vi "FPGA_SviTockovi.vi"() -> ()   [LabVIEW 2014]
uses:
  <vilib>/rvi/Emulation/niFpgaGetClockAttributes.vi
  <vilib>/rvi/Emulation/niFpgaSctlEmulationGetInTimedLoop.vi
  <vilib>/rvi/Emulation/niFpgaEmulationReportErrorSimple.vi
  <vilib>/rvi/eio/common/nirviEmuTemplateMethod_errors.vi
  <vilib>/rvi/Emulation/niFpgaCriticalErrorInLSC.vi
  <vilib>/eio/EIONode/EIONode.xnode
panel:
  in  "stop":bool
  in  "step":sgl(knob) scale=0.0..300.0
  in  "rezolucija":i32(listbox)
  in  "pokreni":bool
  in  "dir 4":bool
  in  "dir 3":bool
  in  "dir 2":bool
  in  "dir 1":bool
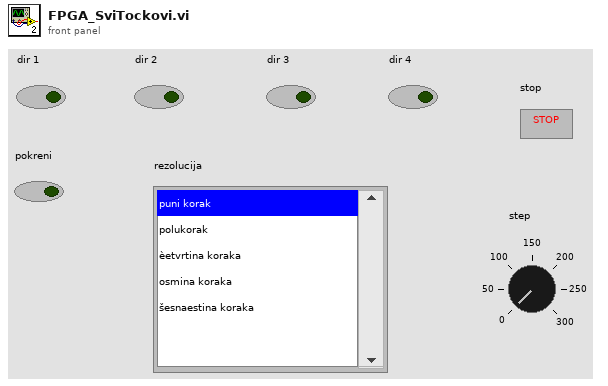
[diagram p1: front panel]
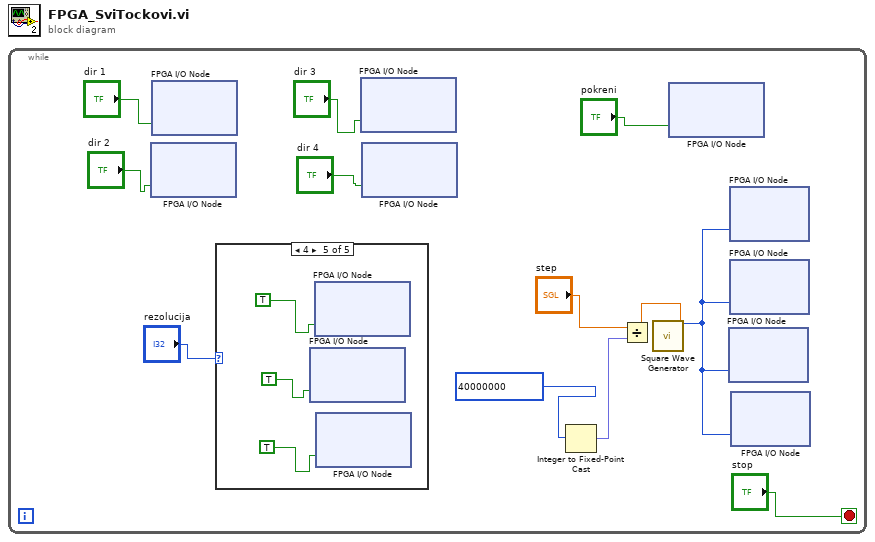
[diagram p0: block diagram]
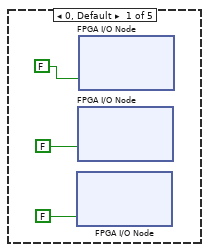
[diagram p2: hidden frame]
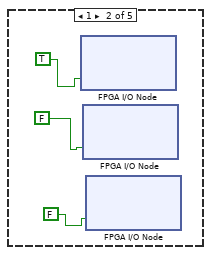
[diagram p3: hidden frame]
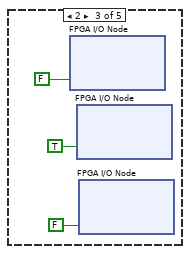
[diagram p4: hidden frame]
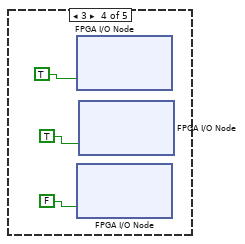
[diagram p5: hidden frame]
diagram:
  n1 = while {
    stop <- "stop" stop-if-true
    n2 = xnode "FPGA I/O Node"("DIO7"="dir 2") -> ()  [unwired: 1 in, 1 out]
    n3 = xnode "FPGA I/O Node"("DIO4"="dir 1") -> ()  [unwired: 1 in, 1 out]
    n4 = case shown="4" "rezolucija" {
      frame 0, Default {
        n5 = xnode "FPGA I/O Node"("DIO22"=FALSE) -> ()  [unwired: 1 in, 1 out]
        n6 = xnode "FPGA I/O Node"("DIO19"=FALSE) -> ()  [unwired: 1 in, 1 out]
        n7 = xnode "FPGA I/O Node"("DIO16"=FALSE) -> ()  [unwired: 1 in, 1 out]
      }
      frame 1 {
        n8 = xnode "FPGA I/O Node"("DIO16"=TRUE) -> ()  [unwired: 1 in, 1 out]
        n9 = xnode "FPGA I/O Node"("DIO19"=FALSE) -> ()  [unwired: 1 in, 1 out]
        n10 = xnode "FPGA I/O Node"("DIO22"=FALSE) -> ()  [unwired: 1 in, 1 out]
      }
      frame 2 {
        n11 = xnode "FPGA I/O Node"("DIO16"=FALSE) -> ()  [unwired: 1 in, 1 out]
        n12 = xnode "FPGA I/O Node"("DIO19"=TRUE) -> ()  [unwired: 1 in, 1 out]
        n13 = xnode "FPGA I/O Node"("DIO22"=FALSE) -> ()  [unwired: 1 in, 1 out]
      }
      frame 3 {
        n14 = xnode "FPGA I/O Node"("DIO16"=TRUE) -> ()  [unwired: 1 in, 1 out]
        n15 = xnode "FPGA I/O Node"("DIO22"=FALSE) -> ()  [unwired: 1 in, 1 out]
        n16 = xnode "FPGA I/O Node"("DIO19"=TRUE) -> ()  [unwired: 1 in, 1 out]
      }
      frame 4 {
        n17 = xnode "FPGA I/O Node"("DIO19"=TRUE) -> ()  [unwired: 1 in, 1 out]
        n18 = xnode "FPGA I/O Node"("DIO16"=TRUE) -> ()  [unwired: 1 in, 1 out]
        n19 = xnode "FPGA I/O Node"("DIO21"=TRUE) -> ()  [unwired: 1 in, 1 out]
      }
    }
    n20 = xnode "FPGA I/O Node"("DIO10"="dir 3") -> ()  [unwired: 1 in, 1 out]
    n21 = xnode "FPGA I/O Node"("DIO13"="dir 4") -> ()  [unwired: 1 in, 1 out]
    n22 = Integer to Fixed-Point Cast(integer=40000000) -> (fixed-point=w11:fxp<+/-,32,32>)  [unwired: 1 in]
    n23 = Divide(x="step", y=w11) -> (x/y=w10:sgl)
    n24 = call "Square Wave Generator"("frequency (periods/tick)"=w10) -> ("square wave out"=w8:i16)  [unwired: 14 in]
    n25 = xnode "FPGA I/O Node"("DIO27"="pokreni") -> ()  [unwired: 1 in, 1 out]
    n26 = xnode "FPGA I/O Node"("AO2"=w8) -> ()  [unwired: 1 in, 1 out]
    n27 = xnode "FPGA I/O Node"("AO0"=w8) -> ()  [unwired: 1 in, 1 out]
    n28 = xnode "FPGA I/O Node"("AO1"=w8) -> ()  [unwired: 1 in, 1 out]
    n29 = xnode "FPGA I/O Node"("AO3"=w8) -> ()  [unwired: 1 in, 1 out]
  }
